vi "Main - On Load.vi"(8 "error in (no error)":errorcluster, 11 "Device Item Ref in":T1 format="%.0x") -> (0 "error out":errorcluster, 3 "Device Item Ref out":T1 format="%.0x")   [LabVIEW 2011, in "Switch-DMM Custom Device.lvlib"]
uses:
  Switch-DMM Custom Device.lvlib
  <vilib>/NI Veristand/Custom Device API/Custom Device Item Ref.ctl
  Controls/Globals.vi
  <vilib>/NI Veristand/Custom Device API/Set Item Property (I32).vi
  <vilib>/NI Veristand/Custom Device API/Custom Device API.lvlib
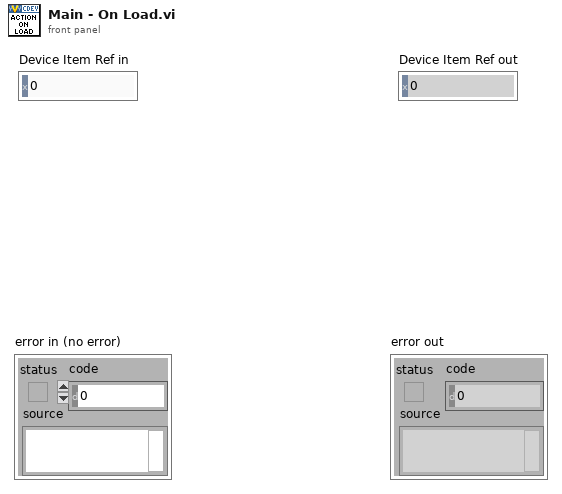
[diagram p1: front panel]
types:
  T1 = typedef "Custom Device API.lvlib/Custom Device Item Ref.ctl" = u64
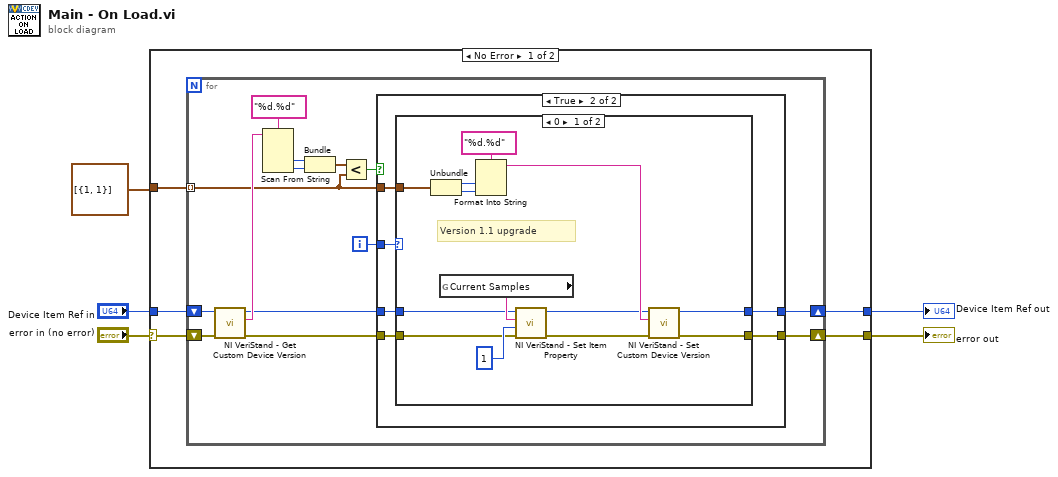
[diagram p0: block diagram]
diagram:
  n1 = case shown="No Error" "error in (no error)" {
    selector: "error in (no error)" -> [w9 w49]
    tunnel: [w6 w49] -> w2
    tunnel: "Device Item Ref in" -> [w8 w48]
    tunnel: [w7 w48] -> w1
    tunnel: cluster{i32, i32}[] [{1, 1}] -> [w10 _]
    frame No Error {
      n2 = for {
        tunnel: w10 -> [w11] mode=indexing
        shift-right: [w15] -> w6
        shift-left: w9 -> [w20]
        shift-right: [w13] -> w7
        shift-left: w8 -> [w19]
        i -> [w12]
        n3 = call <vilib>:"NI VeriStand - Get Custom Device Version.vi"("error in (no error)"=w20, "Device Ref in"=w19) -> ("error out"=w16:errorcluster, "Value"=w18:string, "Device Ref out"=w14:T1)  [unwired: 7 in]
        n4 = Scan From String(format string="%d.%d", input string=w18) -> (output 1=w22:i32, output 2=w23:i32)  [unwired: 4 in, 3 out]
        n5 = Bundle(w22, w23) -> (w24:cluster{i32, i32})  [unwired: 1 in]
        n6 = Less?(x=w24, y=w11) -> (x < y?=w17:bool)
        n7 = case shown="True" w17 {
          tunnel: w16 -> [w26 w32]
          tunnel: [w26 w31] -> w15
          tunnel: w14 -> [w25 w28]
          tunnel: [w25 w29] -> w13
          tunnel: w12 -> [_ w30]
          tunnel: w11 -> [_ w27]
          frame False {
          }
          frame True {
            n8 = case shown="0" w30 {
              tunnel: w32 -> [w35 w47]
              tunnel: [w39 w47] -> w31
              tunnel: [w40 w46] -> w29
              tunnel: w28 -> [w36 w46]
              tunnel: w27 -> [w42 _]
              frame 0 {
                # "Version 1.1 upgrade"
                n9 = Unbundle(w42) -> (w44:i32, w45:i32)
                n10 = global read "Globals.vi" "Current Samples"() -> (w38:string)
                n11 = Format Into String(format string="%d.%d", w44, w45) -> (resulting string=w41:string)  [unwired: 2 in, 1 out]
                n12 = call-poly <vilib>:"NI VeriStand - Set Item Property.vi"("error in (no error)"=w35, "Value"=1, "Property Name"=w38, "Item Ref in"=w36) -> ("error out"=w33:errorcluster, "Item Ref out"=w34:T1)  [unwired: 5 in, 1 out]
                n13 = call <vilib>:"NI VeriStand - Set Custom Device Version.vi"("error in (no error)"=w33, "Value"=w41, "Device Ref in"=w34) -> ("error out"=w39:errorcluster, "Device Ref out"=w40:T1)  [unwired: 7 in]
              }
              frame Default {
              }
            }
          }
        }
      }
    }
    frame Error {
    }
  }
  "error out" <- w2
  "Device Item Ref out" <- w1
